vi "Execute.vi"(8 "error in":errorcluster, 11 "Set Pressure in":refnum<class "Set Pressure.lvclass">) -> (0 "error out":errorcluster, 1 "Next Step?":bool, 2 "MSG":string, 3 "Set Pressure out":refnum<class "Set Pressure.lvclass">)   [LabVIEW 2015, in "Set Pressure.lvclass"]
doc: "Calls the shared variable for the MFC Setpoints and puts in a new value for the pressure setpoint."
uses:
  Set Pressure.lvclass
  Controls/MFC Address.ctl
  Reusable/Sequence/STEPS/LEAVES/Double/Switch DBL.lvclass/Switch DBL.ctl
  Reusable/Sequence/STEPS/LEAVES/Double/Read val.vi
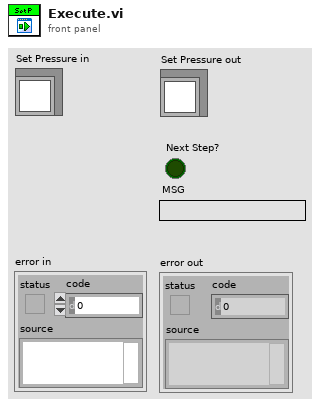
[diagram p1: front panel]
types:
  T1 = typedef "MFC Address.ctl" = enum16{"CRDS Purge", "CRDS Thermodenuded", "CRDS Dry", "CRDS Med RH", "CRDS High RH", "PAS Ch 1", "PAS Ch 2", "PAS Ch3", "PAS Ch 4", "PAS Ch 5", "CLAP", "O3", "Pinlet"}
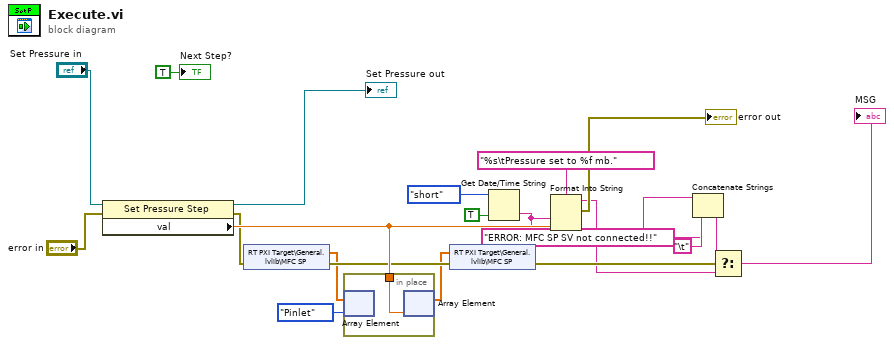
[diagram p0: block diagram]
diagram:
  n1 = property class="Set Pressure Step"(reference="Set Pressure in", error in="error in") -> (reference out=→"Set Pressure out":refnum<class "Set Pressure.lvclass">, error out=w11:errorcluster, "val"=w12:dbl)
  n2 = shared-variable "RT PXI Target\\General.lvlib\\MFC SP"(error in=w11) -> (w7:sgl[], error out=w10:errorcluster)
  n3 = in-place {
    in-place-border: w12 -> [w22]
    n4 = in-place-array #1(w7, MFC_Address."Pinlet" ("Controllers")) -> ()  [unwired: 1 out]
    n5 = in-place-array #1(w22) -> (w8:sgl[])  [unwired: 1 out]
  }
  n6 = shared-variable "RT PXI Target\\General.lvlib\\MFC SP"(w8, error in=w10) -> (error out=w6:errorcluster)
  n7 = Get Date/Time String(date format (0)=enum16{"short", "long", "abbreviated"}."short", want seconds? (F)=TRUE) -> (time string=w4:string)  [unwired: 1 in, 1 out]
  n8 = Format Into String(format string="%s\tPressure set to %f mb.", w4, w12) -> (resulting string=w5:string, error out=→"error out":errorcluster)  [unwired: 2 in]
  n9 = Concatenate Strings(w4, "\t", "ERROR: MFC SP SV not connected!!" ("string")) -> (w2:string)
  n10 = Select(t=w2, s=w6, f=w5) -> (s? t:f=→"MSG":string)
  "Next Step?" <- TRUE ("Next Step?")
